vi "Tester.vi"() -> ()   [LabVIEW 2016, in "Assert API Components.lvlib" / "Assert Service.lvlib" / "UDP Link.lvlib"]
uses:
  UDP Link.lvlib
  UDP Link/UDP Link.lvclass
  C:/Program Files (x86)/National Instruments/LabVIEW 2016/vi.lib/ActorFramework/Actor/Actor.lvclass
  <vilib>/ActorFramework/Actor/Actor.lvclass
panel:
  out "error out":errorcluster
  in  "Port Number":u16
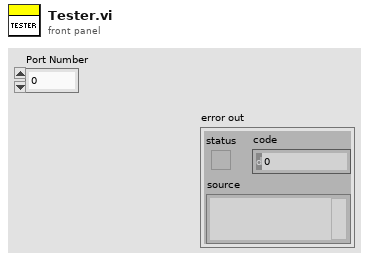
[diagram p1: front panel]
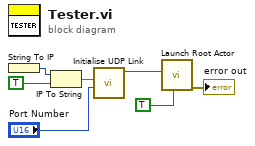
[diagram p0: block diagram]
diagram:
  n1 = String To IP() -> (0:w1:u32)  [unwired: 1 in]
  n2 = IP To String(1:TRUE ("dot notation? (F)"), 2:w1) -> (0:w3:string)
  n3 = call "Initialise UDP Link.vi"("Port Number"="Port Number", "IP Address"=w3) -> ("UDP Link out"=w7:refnum<class "UDP Link.lvclass">)  [unwired: 9 in]
  n4 = call <vilib>:"Launch Root Actor.vi"("Open Actor Core front panel? (F)"=TRUE, "Actor"=w7) -> ("error out"=→"error out":errorcluster)  [unwired: 8 in, 1 out]
